vi "Get Images Per DMA.vi"(11 "images":u32) -> (2 "function return":u32, 3 "images out":u32)   [LabVIEW 2018, in "Copy of Andor SDK.lvlib"]
doc: "EXPNETTYPE unsigned int WINAPI GetImagesPerDMA(unsigned long * images);"
uses:
  Copy of Andor SDK.lvlib
  <userlib>/Andor SDK/ATMCD32D.dll
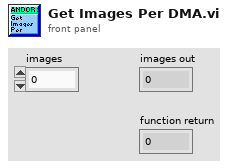
[diagram p1: front panel]
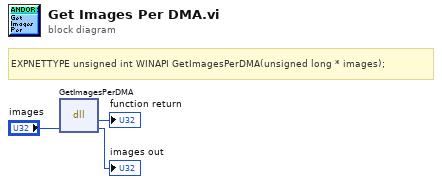
[diagram p0: block diagram]
diagram:
  # "EXPNETTYPE unsigned int WINAPI GetImagesPerDMA(unsigned long * images);"
  n1 = dll-call lib="C:/Program Files (x86)/National Instruments/LabVIEW 2018/user.lib/Andor SDK/ATMCD32D.*" fn="GetImagesPerDMA"("images"="images") -> (→"function return":u32, "images"=→"images out":u32)  [unwired: 3 in, 2 out]
